vi "Digital Tach Process.vi"(5 "reset? (True)":bool=TRUE, 8 "avg on n pulses (1:no average)":i32=1, 9 "pulse/revolution (1)":i32=1, 11 "digital tach info":T1={"tacho counts"=[], "counter timebase [Hz]"=20000000.0, "counter task type"=enum."event counting", "counter digit (32)"=32}) -> (0 "error out":errorcluster, 1 "pulse positions [s]":dbl[](array[numeric]) format="%.2f", 3 "speed profile":T2 {"speed [RPM]" format="%.2f"; "time [s]" format="%.2f"})   [LabVIEW 2017]
doc: "Processes tachometer signals using a digital counter."
uses:
  <vilib>/addons/Sound and Vibration/Order Analysis/Tach Process/SubVIs/digital tach info.ctl
  <vilib>/addons/Sound and Vibration/Order Analysis/Tach Process/SubVIs/speed profile.ctl
  <vilib>/addons/Sound and Vibration/Order Analysis/Tach Process/SoundVib_TachProcess.lvlib
panel:
  # "Digital Tach Process"
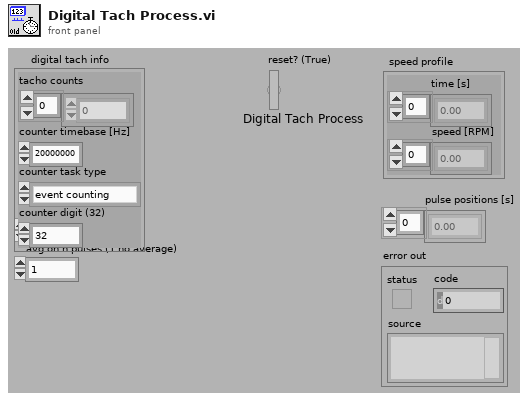
[diagram p1: front panel]
types:
  T1 = typedef "SoundVib_TachProcess.lvlib/digital tach info.ctl" = cluster{"tacho counts":i64[], "counter timebase [Hz]":dbl, "counter task type":enum16{"period measurement", "event counting"}, "counter digit (32)":i32}
  T2 = typedef "SoundVib_TachProcess.lvlib/speed profile.ctl" = cluster{"time [s]":dbl[], "speed [RPM]":dbl[]}
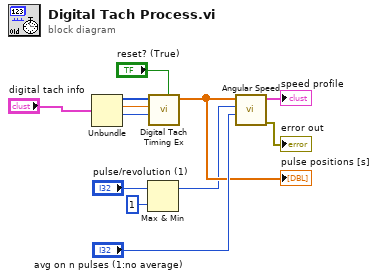
[diagram p0: block diagram]
diagram:
  n1 = Unbundle("digital tach info") -> ("tacho counts"=w6:i64[], "counter timebase [Hz]"=w5:dbl, "counter task type"=w9:enum16{"period measurement", "event counting"})  [unwired: 1 out]
  n2 = Max & Min(x="pulse/revolution (1)", y=1) -> (max(x,y)=w2:i32)  [unwired: 1 out]
  n3 = call <vilib>:"Digital Tach Timing Ex.vi"("reset? (True)"="reset? (True)", "counter task type"=w9, "counter timebase [Hz]"=w5, "tach counts"=w6) -> ("pulse positions [s]"=w8:dbl[])  [unwired: 6 in, 1 out]
  "pulse positions [s]" <- w8
  n4 = call <vilib>:"Angular Speed.vi"("avg on n pulses (1:no average)"="avg on n pulses (1:no average)", "pulse/revolution (1)"=w2, "pulse positions [s]"=w8) -> ("error out"=→"error out":errorcluster, "speed profile"=→"speed profile":T2)  [unwired: 3 in]
